vi "SSI_Close.vi"(4 "Error in (no error)":errorcluster caption="error out（no error）", 6 "Connection ID in":refnum<k5>, 7 "VISA resource name":refnum<visa-resource-name>) -> (0 "Error out":errorcluster caption="error out")   [LabVIEW 2011]
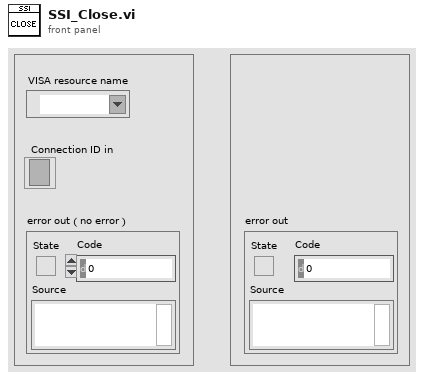
[diagram p1: front panel]
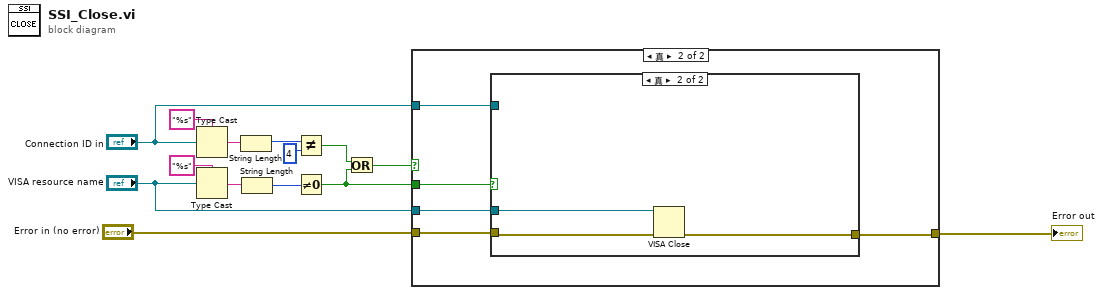
[diagram p0: block diagram]
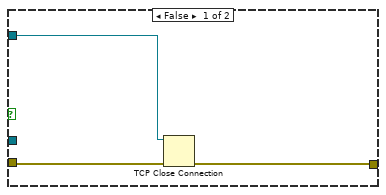
[diagram p3: hidden frame]
diagram:
  n1 = Type Cast(type="%s" ("类型"), x="Connection ID in") -> (*(type *) &x=w12:string)
  n2 = Type Cast(type="%s" ("类型"), x="VISA resource name") -> (*(type *) &x=w11:string)
  n3 = String Length(string=w12) -> (length=w4:i32)
  n4 = String Length(string=w11) -> (length=w10:i32)
  n5 = Not Equal?(x=w4, y=4) -> (x != y?=w9:bool)
  n6 = Not Equal To 0?(x=w10) -> (x != 0?=w7:bool)
  n7 = Or(x=w9, y=w7) -> (x .or. y?=w8:bool)
  n8 = case shown="真" w8 {
    tunnel: [w15 w18] -> w1
    tunnel: "Error in (no error)" -> [w15 w19]
    tunnel: w7 -> [_ w20]
    tunnel: "VISA resource name" -> [_ w17]
    tunnel: "Connection ID in" -> [_ w16]
    frame False {
    }
    frame True {
      n9 = case shown="真" w20 {
        tunnel: w19 -> [w22 w24]
        tunnel: [w23 w26] -> w18
        tunnel: w17 -> [_ w25]
        tunnel: w16 -> [w21 _]
        frame False {
          n10 = TCP Close Connection(connection ID=w21, error in (no error)=w22) -> (error out=w23:errorcluster)  [unwired: 1 in, 1 out]
        }
        frame True {
          n11 = VISA Close(VISA resource name=w25, error in (no error)=w24) -> (error out=w26:errorcluster)
        }
      }
    }
  }
  "Error out" <- w1
